vi "Robot Global Data.vi"() -> ()   [LabVIEW 2011]
doc: "This global VI can contain as many global variables as you need. Place a control on the panel, give it a good name. To read or write to it from a VI, drag the icon to the diagram of that VI. You can also drag from the project. Click on the node to change which global you access. You shouldn't have multiple locations writing to a global or it will cause a race-condition."
uses:
  <vilib>/Rock Robotics/WPI/Camera/WPI_CameraImageSize.ctl
panel:
  in  "R Joystick Button 8":bool
  in  "R Joystick Button 7":bool
  in  "R Joystick Button 6":bool
  in  "R Joystick Button 5":bool
  in  "R Joystick Button 4":bool
  in  "R Joystick Button 3":bool
  in  "R Joystick Button 2":bool
  in  "R Joystick Button 1":bool
  in  "L Joystick Button 8":bool
  in  "L Joystick Button 7":bool
  in  "L Joystick Button 6":bool
  in  "L Joystick Button 5":bool
  in  "L Joystick Button 4":bool
  in  "L Joystick Button 3":bool
  in  "L Joystick Button 2":bool
  in  "L Joystick Button 1":bool
  in  "LED toggle rate (ms)":u32=20
  in  "image size":T1=enum."320x240"
  in  "Enable Vision":bool
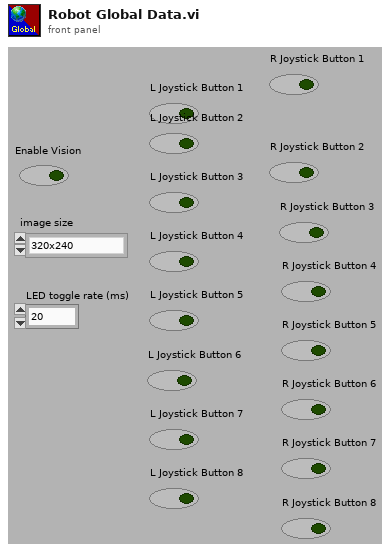
[diagram p1: front panel]
types:
  T1 = typedef "WPI_CameraImageSize.ctl" = enum16{"640x480", "320x240", "160x120"}
diagram:
